vi "Get Checksum.vi"(8 "error in (no error)":errorcluster, 11 "System in":refnum<k21>) -> (0 "error out":errorcluster, 2 "Checksum":u32, 3 "System out":refnum<k21>)   [LabVIEW 2012, in "nisyscfg.lvlib"]
uses:
  <vilib>/nisyscfg/nisyscfg.lvlib
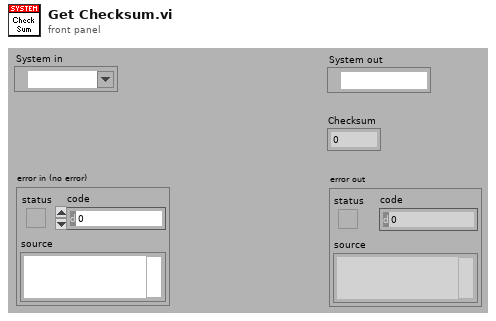
[diagram p1: front panel]
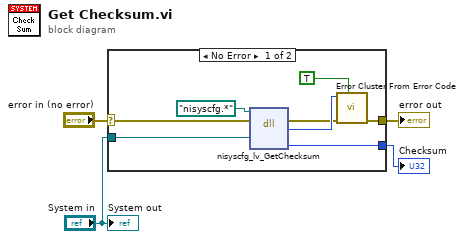
[diagram p0: block diagram]
diagram:
  n1 = case shown="No Error" "error in (no error)" {
    selector: "error in (no error)" -> [w10 w13]
    tunnel: "System in" -> [w12 _]
    tunnel: [w11 _] -> w4
    tunnel: [w6 w13] -> w2
    frame No Error {
      n2 = dll-call lib="nisyscfg.*" fn="nisyscfg_lv_GetChecksum" label="GetChecksum"(path in=path "nisyscfg.*", error in=w10, "session"=w12) -> (error out=w7:errorcluster, "result"=w8:i32, "checksum"=w11:u32)  [unwired: 3 in, 1 out]
      n3 = call <vilib>:"Error Cluster From Error Code.vi"("show call chain? (False)"=TRUE, "error in (no error)"=w7, "error code (0)"=w8) -> ("error out"=w6:errorcluster)  [unwired: 6 in]
    }
    frame Error {
    }
  }
  "error out" <- w2
  "Checksum" <- w4
  "System out" <- "System in"
